vi "Ballard - Arinc-429 - Clear Parameters_old.vi"(8 "error in (no error)":errorcluster, 11 "Node Ptr":u64 format="%.0x") -> (0 "error out":errorcluster)   [LabVIEW 2017]
uses:
  Shared/Controls and Global/Global.vi
  <vilib>/NI Veristand/Custom Device Tools/Custom Device Utility Library/NI VeriStand - Search for All Items by GUID.vi
  <vilib>/NI Veristand/Custom Device API/Custom Device API.lvlib
  Shared/Ballard Arinc-429 Shared.lvlib
  <vilib>/NI Veristand/Custom Device Tools/Custom Device Utility Library/Custom Device Utility Library.lvlib
  <vilib>/NI Veristand/Custom Device Tools/Custom Device Utility Library/NI VeriStand - Search for Item by GUID.vi
panel:
  in  "Tag":string
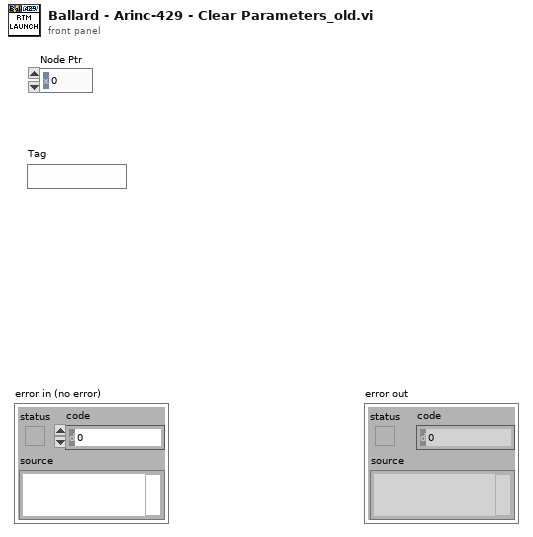
[diagram p1: front panel]
types:
  T1 = typedef "Custom Device API.lvlib/Custom Device Item Ref.ctl" = u64
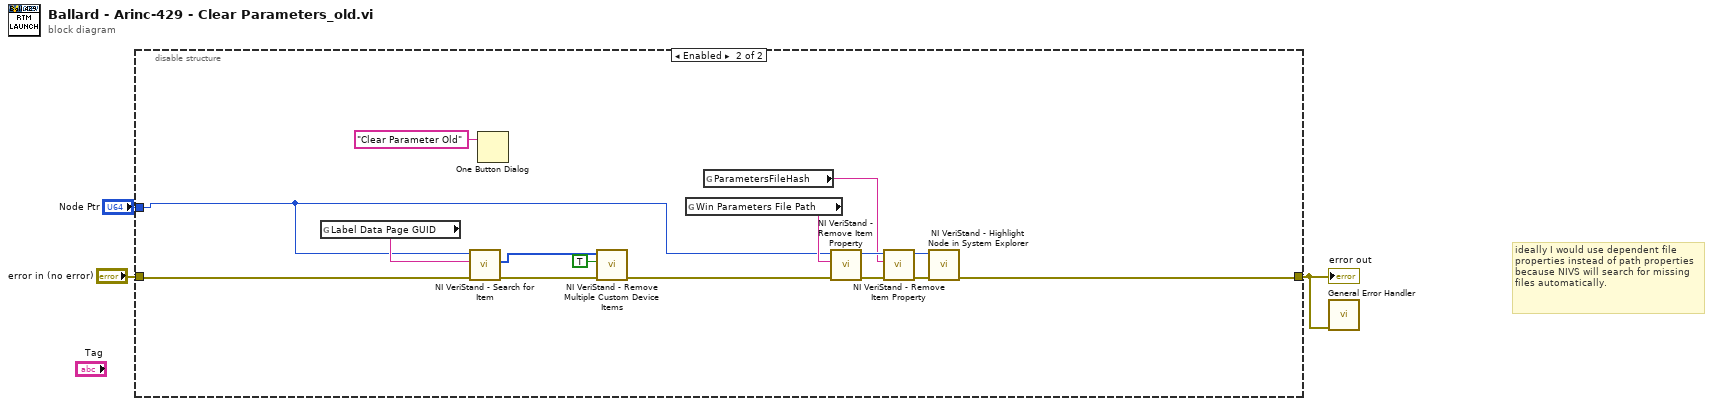
[diagram p0: block diagram]
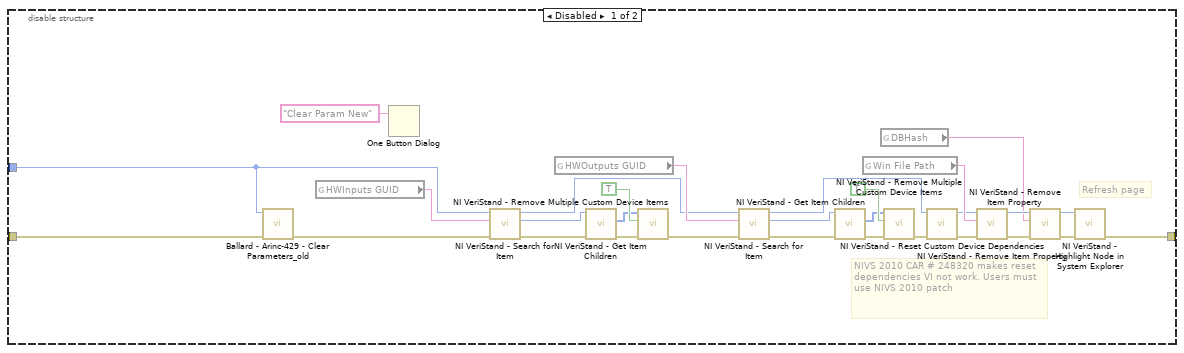
[diagram p2: hidden frame]
diagram:
  # "ideally I would use dependent file properties instead of path properties because NIVS will search for missing files automatically."
  n1 = disable-structure shown="Enabled" {
    disable-tunnel: [w13 w35] -> w3
    disable-tunnel: "error in (no error)" -> [w7 w37]
    disable-tunnel: "Node Ptr" -> [w5 w36]
    frame Disabled {
      # "NIVS 2010 CAR # 248320 makes reset dependencies VI not work. Users must use NIVS 2010 patch"
      # "Refresh page"
      n2 = call "Ballard - Arinc-429 - Clear Parameters_old.vi"("error in (no error)"=w7, "Node Ptr"=w5) -> ("error out"=w6:errorcluster)  [unwired: 9 in]
      n3 = global read "Global.vi" "HWInputs GUID"() -> (w26:string)
      n4 = One Button Dialog(message="Clear Param New") -> ()  [unwired: 1 in, 1 out]
      n5 = call-poly <vilib>:"NI VeriStand - Search for Item.vi"("error in"=w6, "Item GUID"=w26, "Section Ref in"=w5) -> ("error out"=w22:errorcluster, "Item Ref"=w25:T1, "Section Ref out"=w15:T1)  [unwired: 5 in, 1 out]
      n6 = global read "Global.vi" "HWOutputs GUID"() -> (w20:string)
      n7 = call <vilib>:"NI VeriStand - Get Item Children.vi"("error in (no error)"=w22, "Item Ref in"=w25) -> ("error out"=w32:errorcluster, "Child Refs"=w27:T1[])  [unwired: 6 in, 2 out]
      n8 = call <vilib>:"NI VeriStand - Remove Multiple Custom Device Items.vi"("error in (no error)"=w32, "Force Delete (F)"=TRUE, "Item Refs in"=w27) -> ("error out"=w21:errorcluster)  [unwired: 7 in, 1 out]
      n9 = call-poly <vilib>:"NI VeriStand - Search for Item.vi"("error in"=w21, "Item GUID"=w20, "Section Ref in"=w15) -> ("error out"=w18:errorcluster, "Item Ref"=w19:T1, "Section Ref out"=w14:T1)  [unwired: 5 in, 1 out]
      n10 = call <vilib>:"NI VeriStand - Get Item Children.vi"("error in (no error)"=w18, "Item Ref in"=w19) -> ("error out"=w23:errorcluster, "Child Refs"=w17:T1[])  [unwired: 6 in, 2 out]
      n11 = global read "Global.vi" "Win File Path"() -> (w29:string)
      n12 = global read "Global.vi" "DBHash"() -> (w8:string)
      n13 = call <vilib>:"NI VeriStand - Remove Multiple Custom Device Items.vi"("error in (no error)"=w23, "Force Delete (F)"=TRUE, "Item Refs in"=w17) -> ("error out"=w16:errorcluster)  [unwired: 7 in, 1 out]
      n14 = call <vilib>:"NI VeriStand - Reset Custom Device Dependencies.vi"("error in (no error)"=w16, "Device Ref in"=w14) -> ("error out"=w30:errorcluster, "Device Ref out"=w28:T1)  [unwired: 8 in]
      n15 = call <vilib>:"NI VeriStand - Remove Item Property.vi"("error in (no error)"=w30, "Property Name"=w29, "Item Ref in"=w28) -> ("error out"=w12:errorcluster, "Item Ref out"=w11:T1)  [unwired: 6 in, 1 out]
      n16 = call <vilib>:"NI VeriStand - Remove Item Property.vi"("error in (no error)"=w12, "Property Name"=w8, "Item Ref in"=w11) -> ("error out"=w10:errorcluster, "Item Ref out"=w9:T1)  [unwired: 6 in, 1 out]
      n17 = call <vilib>:"NI VeriStand - Highlight Node in System Explorer.vi"("error in (no error)"=w10, "Item Ref in"=w9) -> ("error out"=w13:errorcluster)  [unwired: 8 in, 1 out]
    }
    frame Enabled {
      n18 = global read "Global.vi" "Label Data Page GUID"() -> (w41:string)
      n19 = call-poly <vilib>:"NI VeriStand - Search for Item.vi"("error in"=w37, "Item GUID"=w41, "Section Ref in"=w36) -> ("error out"=w40:errorcluster, "Item Refs"=w38:T1[])  [unwired: 5 in, 2 out]
      n20 = One Button Dialog(message="Clear Parameter Old") -> ()  [unwired: 1 in, 1 out]
      n21 = call <vilib>:"NI VeriStand - Remove Multiple Custom Device Items.vi"("error in (no error)"=w40, "Force Delete (F)"=TRUE, "Item Refs in"=w38) -> ("error out"=w34:errorcluster)  [unwired: 7 in, 1 out]
      n22 = global read "Global.vi" "Win Parameters File Path"() -> (w47:string)
      n23 = global read "Global.vi" "ParametersFileHash"() -> (w42:string)
      n24 = call <vilib>:"NI VeriStand - Remove Item Property.vi"("error in (no error)"=w34, "Property Name"=w47, "Item Ref in"=w36) -> ("error out"=w46:errorcluster, "Item Ref out"=w45:T1)  [unwired: 6 in, 1 out]
      n25 = call <vilib>:"NI VeriStand - Remove Item Property.vi"("error in (no error)"=w46, "Property Name"=w42, "Item Ref in"=w45) -> ("error out"=w44:errorcluster, "Item Ref out"=w43:T1)  [unwired: 6 in, 1 out]
      n26 = call <vilib>:"NI VeriStand - Highlight Node in System Explorer.vi"("error in (no error)"=w44, "Item Ref in"=w43) -> ("error out"=w35:errorcluster)  [unwired: 8 in, 1 out]
    }
  }
  "error out" <- w3
  n27 = call <vilib>:"General Error Handler.vi"("error in (no error)"=w3) -> ()  [unwired: 10 in, 5 out]
